vi "Kill CCD-PDA Exposure.vi"   [LabVIEW 2019]
uses:
  Globals and TypeDefs/Type Definitions.llb/3 way Status.ctl
  IGA3000/IGA_comm.llb/Comm Params.ctl
  Globals and TypeDefs/gStatus.vi
types:
  T1 = typedef "3 way Status.ctl" = u8
  T2 = typedef "Comm Params.ctl" = cluster{"Comm Interface":u16, "BUS":i16, "Address":i16, "Com Port":i32}
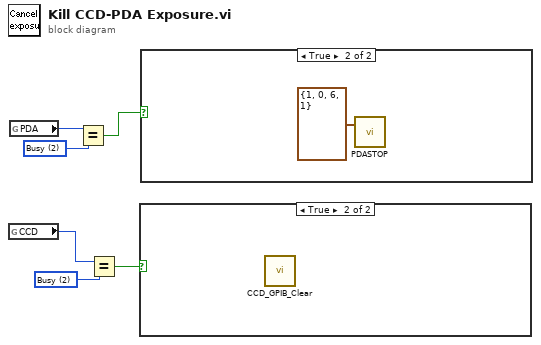
[diagram p0: block diagram]
diagram:
  w3 = T1 2 items=["N.A.", "OK", "Busy", "Done"] ("y")
  w5 = T1 2 items=["N.A.", "OK", "Busy", "Done"] ("y")
  n1 = global read "gStatus.vi" "CCD"() -> (w2:T1)
  n2 = global read "gStatus.vi" "PDA"() -> (w6:T1)
  n3 = Equal?(x=w6, y=w5) -> (x = y?=w4:bool)
  n4 = Equal?(x=w2, y=w3) -> (x = y?=w1:bool)
  n5 = case shown="True" w1 {
    frame False {
    }
    frame True {
      n6 = call "CCD_GPIB_Clear.vi"() -> ()  [unwired: 5 in, 1 out]
    }
  }
  n7 = case shown="True" w4 {
    frame False {
    }
    frame True {
      n8 = call "PDASTOP.VI"("Comm Params"=T2 {"Comm Interface"=1, "BUS"=0, "Address"=6, "Com Port"=1}) -> ()  [unwired: 1 in, 2 out]
    }
  }
